vi "open image.vi"(11 "image path":path) -> (0 "error out":errorcluster, 2 "image data":T1)   [LabVIEW 2009]
uses:
  <vilib>/picture/picture.llb/imagedata.ctl
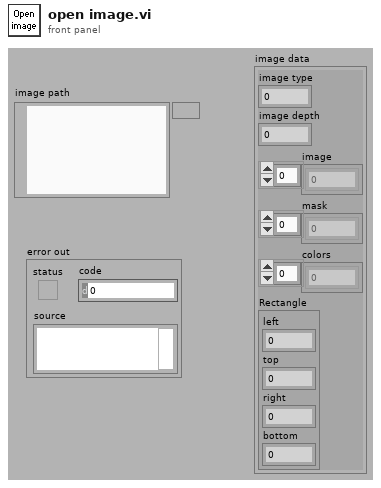
[diagram p1: front panel]
types:
  T1 = typedef "imagedata.ctl" = cluster{"image type":i32, "image depth":i32, "image":u8[], "mask":u8[], "colors":u32[], "Rectangle":cluster{"left":i16, "top":i16, "right":i16, "bottom":i16}}
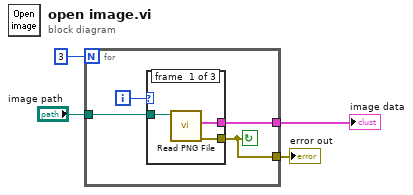
[diagram p0: block diagram]
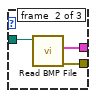
[diagram p2: hidden frame]
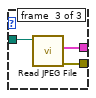
[diagram p3: hidden frame]
diagram:
  n1 = for {
    N: 3 -> [_]
    tunnel: "image path" -> [w7]
    tunnel: [w6] -> w1
    tunnel: [w5] -> w2
    i -> [w8]
    stop <- w5 continue-if-true
    n2 = case shown="2" w8 {
      tunnel: w7 -> [w11 w14 w17]
      tunnel: [w10 w13 w16] -> w6
      tunnel: [w9 w12 w15] -> w5
      frame #0 {
        n3 = call <vilib>:"Read PNG File.vi"("path to PNG file"=w11) -> ("error out"=w9:errorcluster, "image data"=w10:T1)  [unwired: 8 in, 1 out]
      }
      frame #1 {
        n4 = call <vilib>:"Read BMP File.vi"("path to BMP file"=w14) -> ("error out"=w12:errorcluster, "image data"=w13:T1)  [unwired: 8 in, 1 out]
      }
      frame #2 {
        n5 = call <vilib>:"Read JPEG File.vi"("path to JPEG file"=w17) -> ("error out"=w15:errorcluster, "image data"=w16:T1)  [unwired: 8 in, 1 out]
      }
    }
  }
  "error out" <- w2
  "image data" <- w1
